vi "Read AppEvent Queue.vi"(8 "error in (no error)":errorcluster, 11 "EventLog in":refnum<class "EventLog.lvclass">) -> (0 "error out":errorcluster, 2 "AppEvent Queue":refnum<queue>, 3 "EventLog out":refnum<class "EventLog.lvclass">)   [LabVIEW 2019, in "EventLog.lvlib" / "EventLog.lvclass"]
uses:
  EventLog.lvclass
  Classes/Event/Event.lvclass
  EventLog.lvclass/EventLog.ctl
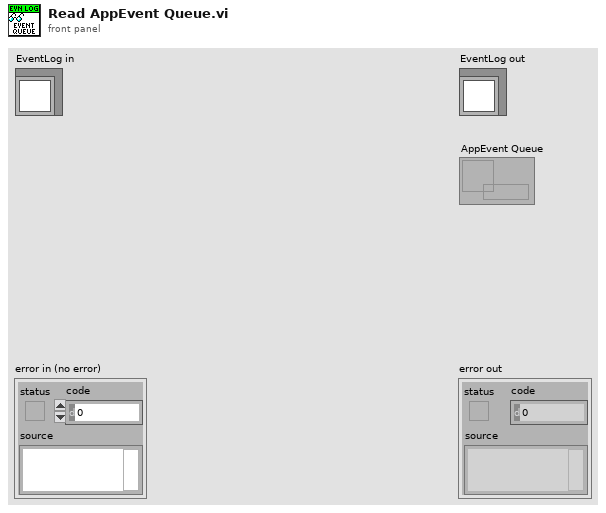
[diagram p1: front panel]
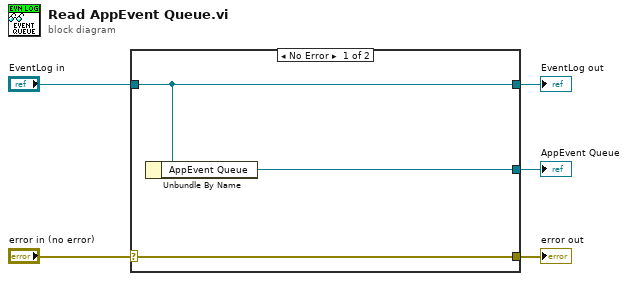
[diagram p0: block diagram]
diagram:
  n1 = case shown="No Error" "error in (no error)" {
    selector: "error in (no error)" -> [w8 w9]
    tunnel: [w8 w9] -> w4
    tunnel: [w7 w10] -> w2
    tunnel: "EventLog in" -> [w7 w10]
    tunnel: [w6 _] -> w1
    frame No Error {
      n2 = Unbundle By Name(w7) -> ("AppEvent Queue"=w6:refnum<queue>)
    }
    frame Error {
    }
  }
  "error out" <- w4
  "EventLog out" <- w2
  "AppEvent Queue" <- w1
